vi "Get Parent Hwnd.vi"(8 "error in (no error)":errorcluster, 11 "Hwnd In":u32) -> (0 "error out":errorcluster, 2 "Parent":i32, 3 "Hwnd Out":u32)   [LabVIEW 2016, in "LV MDI.lvclass"]
doc: "Retrieves Parent window handle of specified window."
uses:
  LV MDI.lvclass
  user32.dll
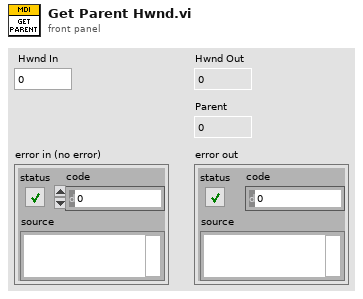
[diagram p1: front panel]
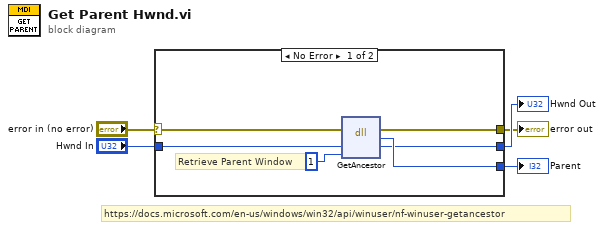
[diagram p0: block diagram]
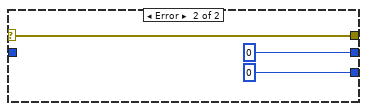
[diagram p2: hidden frame]
diagram:
  # "https://docs.microsoft.com/en-us/windows/win32/api/winuser/nf-winuser-getancestor"
  n1 = case shown="No Error" "error in (no error)" {
    selector: "error in (no error)" -> [w9 w14]
    tunnel: [w11 0 ("Parent")] -> w5
    tunnel: "Hwnd In" -> [w10 _]
    tunnel: [w8 u32 0 ("Hwnd")] -> w2
    tunnel: [w7 w14] -> w1
    frame No Error {
      # "Retrieve Parent Window"
      n2 = dll-call lib="user32.dll" fn="GetAncestor"(error in=w9, "Hwnd"=w10, "gaflags"=1) -> (error out=w7:errorcluster, "Parent"=w11:i32, "Hwnd"=w8:u32)  [unwired: 3 in, 1 out]
    }
    frame Error {
    }
  }
  "Parent" <- w5
  "Hwnd Out" <- w2
  "error out" <- w1
